vi "RUSHClimber.vi"(1 "In Cluster":T2) -> (0 "Out Cluster":T3)   [LabVIEW 2012]
panel:
  out "ClimbConst":T1
  out "ClimbPOTDep":dbl
  out "ClimbManualDep":dbl
  out "ClimbManualExt":dbl
  in  "Extension Speed":dbl=0.75
  in  "Deploy Speed":dbl=0.75
  in  "Deadband":dbl=0.1
  # "For Local use only"
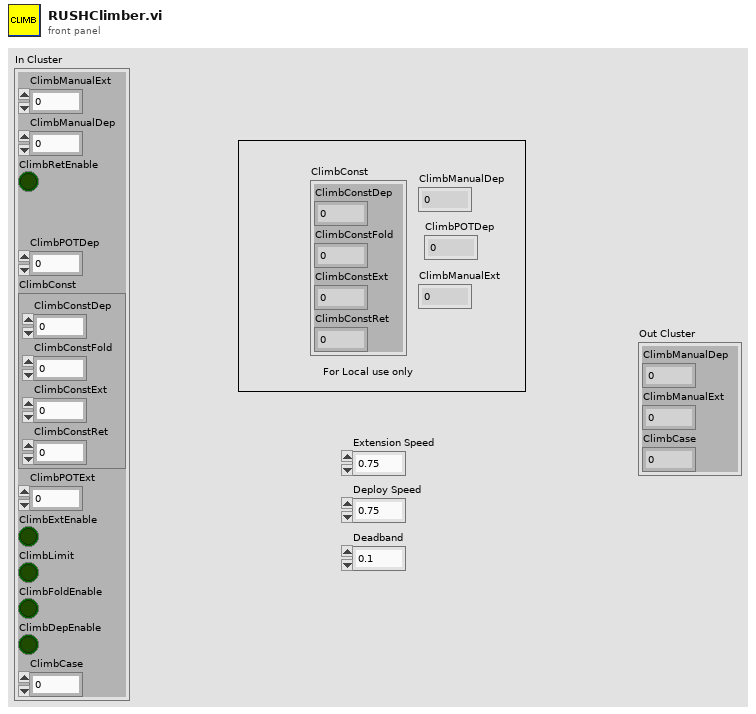
[diagram p1: front panel]
types:
  T1 = cluster{"ClimbConstDep":dbl, "ClimbConstFold":dbl, "ClimbConstExt":dbl, "ClimbConstRet":dbl}
  T2 = cluster{"ClimbManualExt":dbl, "ClimbManualDep":dbl, "ClimbRetEnable":bool, "ClimbPOTDep":dbl, "ClimbConst":cluster{"ClimbConstDep":dbl, "ClimbConstFold":dbl, "ClimbConstExt":dbl, "ClimbConstRet":dbl}, "ClimbPOTExt":dbl, "ClimbExtEnable":bool, "ClimbLimit":bool, "ClimbFoldEnable":bool, "ClimbDepEnable":bool, "ClimbCase":dbl}
  T3 = cluster{"ClimbManualDep":dbl, "ClimbManualExt":dbl, "ClimbCase":i32}
  T4 = cluster{"ClimbManualDep":dbl, "ClimbManualExt":dbl, "t":i32}
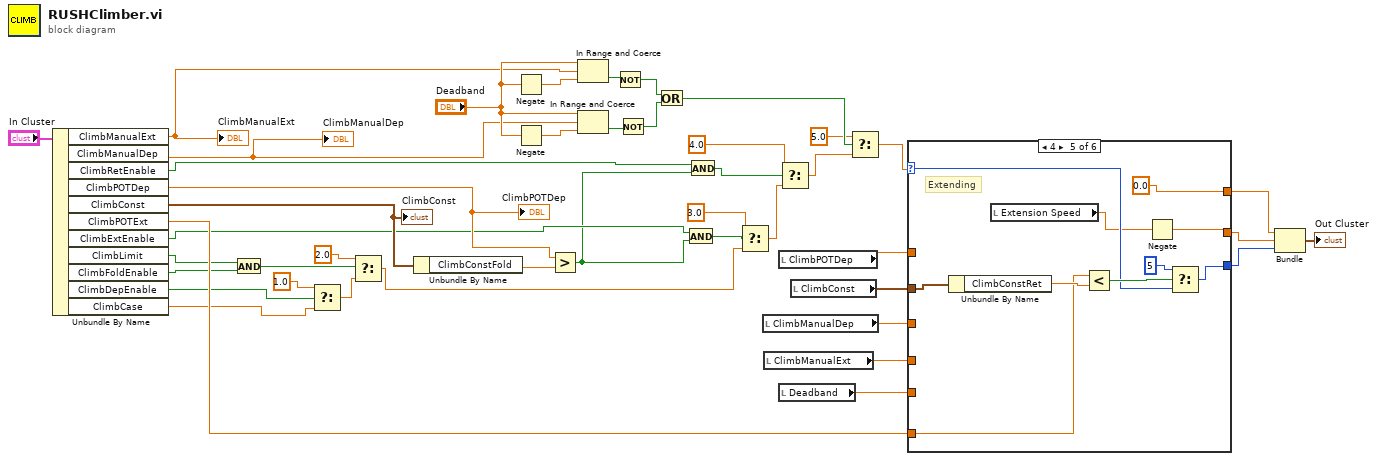
[diagram p0: block diagram]
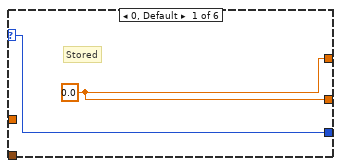
[diagram p2: hidden frame]
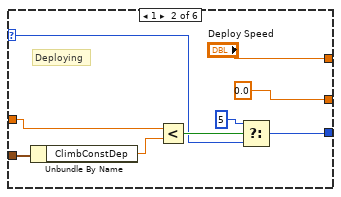
[diagram p3: hidden frame]
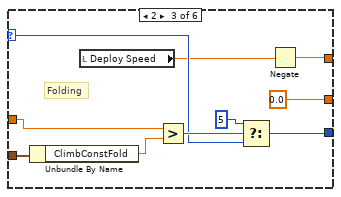
[diagram p4: hidden frame]
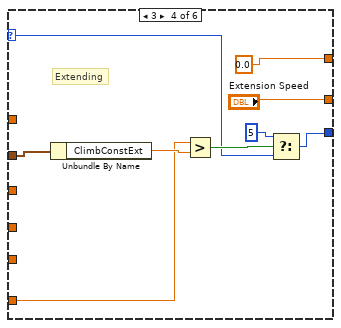
[diagram p5: hidden frame]
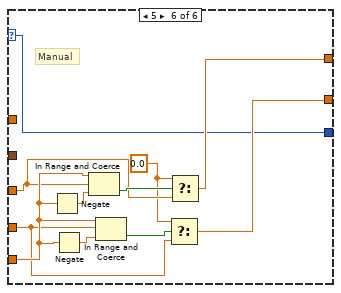
[diagram p6: hidden frame]
diagram:
  n1 = Unbundle By Name("In Cluster") -> ("ClimbManualExt"=w15:dbl, "ClimbManualDep"=w14:dbl, "ClimbRetEnable"=w13:bool, "ClimbPOTDep"=w12:dbl, "ClimbConst"=w11:T1, "ClimbPOTExt"=w10:dbl, "ClimbExtEnable"=w9:bool, "ClimbLimit"=w8:bool, "ClimbFoldEnable"=w7:bool, "ClimbDepEnable"=w4:bool, "ClimbCase"=w6:dbl)
  "ClimbManualExt" <- w15
  "ClimbManualDep" <- w14
  "ClimbPOTDep" <- w12
  "ClimbConst" <- w11
  n2 = And(x=w8, y=w7) -> (x .and. y?=w42:bool)
  n3 = Select(t=1.0, s=w4, f=w6) -> (s? t:f=w41:dbl)
  n4 = Select(t=2.0, s=w42, f=w41) -> (s? t:f=w33:dbl)
  n5 = Unbundle By Name(w11) -> ("ClimbConstFold"=w30:dbl)
  n6 = Negate(x="Deadband") -> (-x=w43:dbl)
  n7 = Negate(x="Deadband") -> (-x=w44:dbl)
  n8 = Greater?(x=w12, y=w30) -> (0:w1:bool)
  n9 = In Range and Coerce(upper limit="Deadband", x=w15, lower limit=w43) -> (In Range?=w26:bool)  [unwired: 1 out]
  n10 = In Range and Coerce(upper limit="Deadband", x=w14, lower limit=w44) -> (In Range?=w27:bool)  [unwired: 1 out]
  n11 = Not(x=w26) -> (.not. x?=w25:bool)
  n12 = Not(x=w27) -> (.not. x?=w24:bool)
  n13 = Or(x=w25, y=w24) -> (x .or. y?=w23:bool)
  n14 = And(x=w9, y=w1) -> (x .and. y?=w39:bool)
  n15 = And(x=w13, y=w1) -> (x .and. y?=w35:bool)
  n16 = Select(t=3.0, s=w39, f=w33) -> (s? t:f=w37:dbl)
  n17 = local read "ClimbManualDep"() -> (w28:dbl)
  n18 = local read "ClimbManualExt"() -> (w22:dbl)
  n19 = local read "ClimbPOTDep"() -> (w31:dbl)
  n20 = local read "Deadband"() -> (w21:dbl)
  n21 = Select(t=4.0, s=w35, f=w37) -> (s? t:f=w3:dbl)
  n22 = local read "ClimbConst"() -> (w29:T1)
  n23 = Select(t=5.0 ("f"), s=w23, f=w3) -> (s? t:f=w32:dbl)
  n24 = case shown="4" w32 {
    selector: w32 -> [w45 w51 w61 w71 w81 w85]
    tunnel: w31 -> [_ w53 w63 _ _ _]
    tunnel: w29 -> [_ w55 w65 w70 w80 _]
    tunnel: [w45 w49 w59 w68 w78 w85] -> w18
    tunnel: [w46 "Deploy Speed" w56 0.0 ("Extend Speed") 0.0 ("Extend Speed") w87] -> w20
    tunnel: [w46 0.0 ("Extend Speed") 0.0 ("Extend Speed") "Extension Speed" w75 w86] -> w19
    tunnel: w28 -> [_ _ _ _ _ w90]
    tunnel: w22 -> [_ _ _ _ _ w88]
    tunnel: w21 -> [_ _ _ _ _ w93]
    tunnel: w10 -> [_ _ _ w69 w79 _]
    frame 0, Default {
      w46 = 0.0
      # "Stored"
    }
    frame 1 {
      # "Deploying"
      n25 = Unbundle By Name(w55) -> ("ClimbConstDep"=w54:dbl)
      n26 = Less?(x=w53, y=w54) -> (x < y?=w52:bool)
      n27 = Select(t=5, s=w52, f=w51) -> (s? t:f=w49:i32)
    }
    frame 2 {
      # "Folding"
      n28 = Unbundle By Name(w65) -> ("ClimbConstFold"=w64:dbl)
      n29 = local read "Deploy Speed"() -> (w57:dbl)
      n30 = Greater?(x=w63, y=w64) -> (0:w62:bool)
      n31 = Select(t=5, s=w62, f=w61) -> (s? t:f=w59:i32)
      n32 = Negate(x=w57) -> (-x=w56:dbl)
    }
    frame 3 {
      # "Extending"
      n33 = Unbundle By Name(w70) -> ("ClimbConstExt"=w74:dbl)
      n34 = Greater?(x=w69, y=w74) -> (0:w73:bool)
      n35 = Select(t=5, s=w73, f=w71) -> (s? t:f=w68:i32)
    }
    frame 4 {
      # "Extending"
      n36 = Unbundle By Name(w80) -> ("ClimbConstRet"=w84:dbl)
      n37 = local read "Extension Speed"() -> (w76:dbl)
      n38 = Less?(x=w79, y=w84) -> (x < y?=w83:bool)
      n39 = Negate(x=w76) -> (-x=w75:dbl)
      n40 = Select(t=5, s=w83, f=w81) -> (s? t:f=w78:i32)
    }
    frame 5 {
      w89 = 0.0 ("t")
      # "Manual"
      n41 = Negate(x=w93) -> (-x=w94:dbl)
      n42 = Negate(x=w93) -> (-x=w95:dbl)
      n43 = In Range and Coerce(upper limit=w93, x=w90, lower limit=w94) -> (In Range?=w91:bool)  [unwired: 1 out]
      n44 = In Range and Coerce(upper limit=w93, x=w88, lower limit=w95) -> (In Range?=w92:bool)  [unwired: 1 out]
      n45 = Select(t=w89, s=w92, f=w88) -> (s? t:f=w86:dbl)
      n46 = Select(t=w89, s=w91, f=w90) -> (s? t:f=w87:dbl)
    }
  }
  n47 = Bundle("ClimbManualDep"=w20, "ClimbManualExt"=w19, "t"=w18) -> (→"Out Cluster":T4)  [unwired: 1 in]
